vi "CAEN PSM SMART HV.vi"() -> ()   [LabVIEW 2017]
uses:
  <instrlib>/CAEN PSM/CAEN PSM.lvlib
panel:
  out "Output values":string[](array[string])
  in  "Value":string
  in  "mon button":bool
  in  "set button":bool
  out "Parameter descriptor":T1
  in  "info button":bool
  out "Connection status":bool
  in  "stop":bool
  in  "OK Button":bool
  out "error out":errorcluster
  in  "Tab Control":enum32{"Board", "Channel"}(tab)
  in  "Board Parameter":string(combo)
  in  "all_ch":bool
  in  "Channel number":u8
  in  "Channel Parameter":string(combo)
  out "Channel Parameters list":string[](array[string])
  out "Board Parameters list":string[](array[string])
  out "Module Info":T2
  in  "VISA resource name":refnum<visa-resource-name>
  # "CAEN PSM for the SMART HV devices\nVI example"
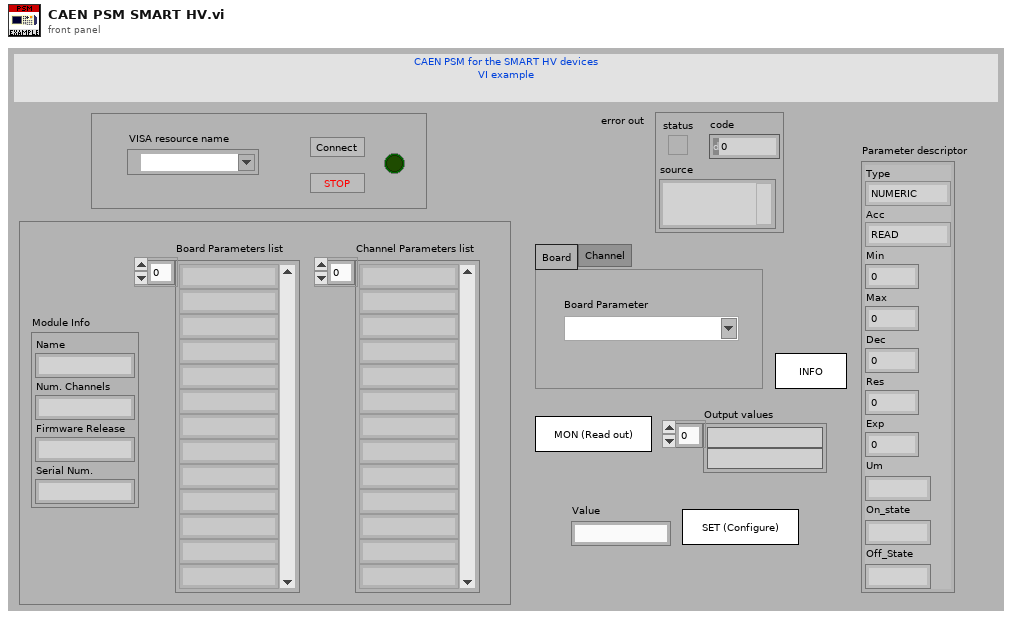
[diagram p1: front panel]
types:
  T1 = cluster{"Type":enum16{"NUMERIC", "ONOFF", "CHSTATUS", "BDSTATUS", "BINARY", "STRING", "ENUM"}, "Acc":enum16{"READ", "WRITE", "READ_WRITE"}, "Min":u32, "Max":u32, "Dec":u32, "Res":u32, "Exp":i32, "Um":string, "On_state":string, "Off_State":string}
  T2 = cluster{"Name":string, "Num. Channels":string, "Firmware Release":string, "Serial Num.":string}
  T3 = typedef "CAEN PSM.lvlib/BoardHandle.ctl" = cluster{"VISA resource name":refnum<visa-resource-name>, "Board address":i8, "NChannels":u8}
  T4 = enum8{"Enabled", "Disabled", "Disabled and Grayed Out"}
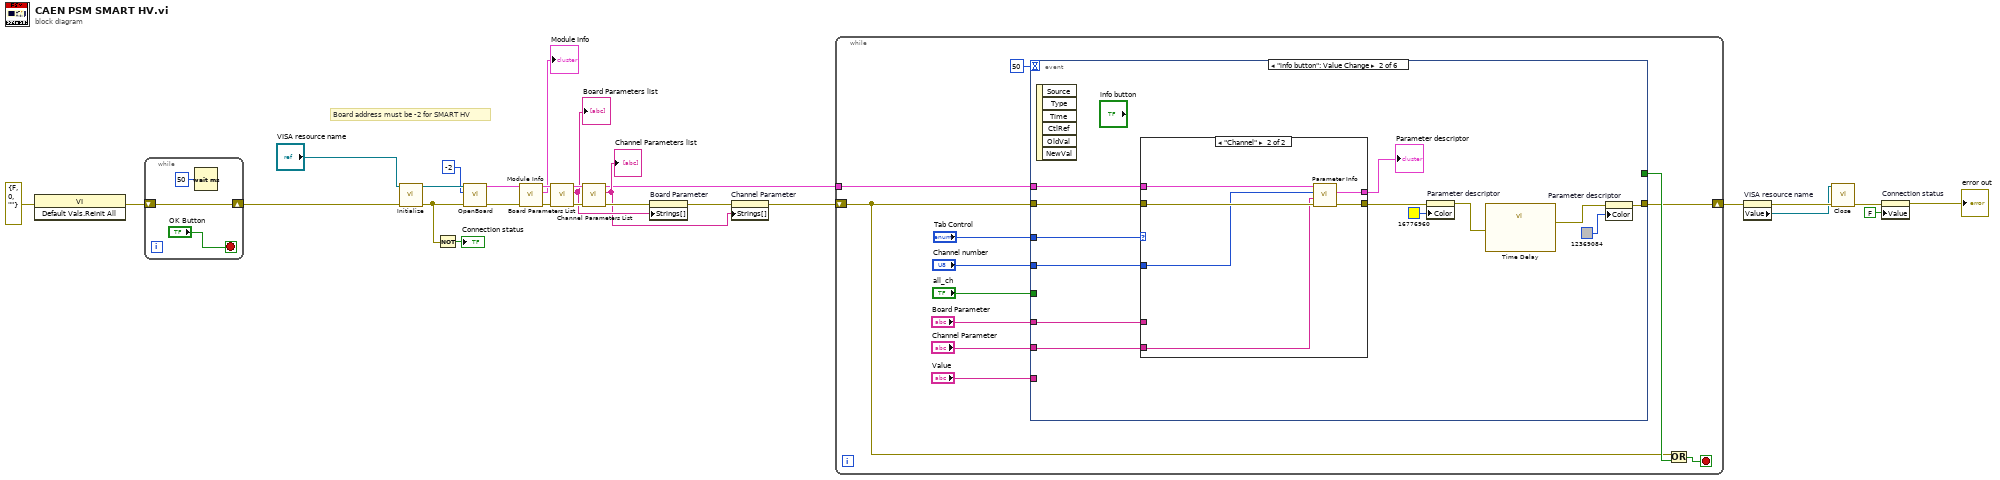
[diagram p0: block diagram]
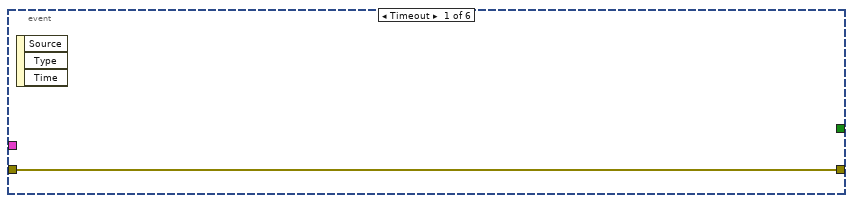
[diagram p2: hidden frame]
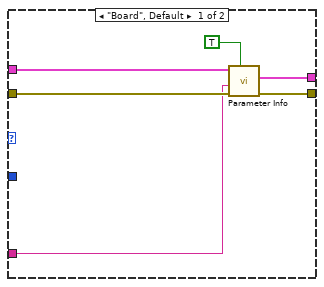
[diagram p3: hidden frame]
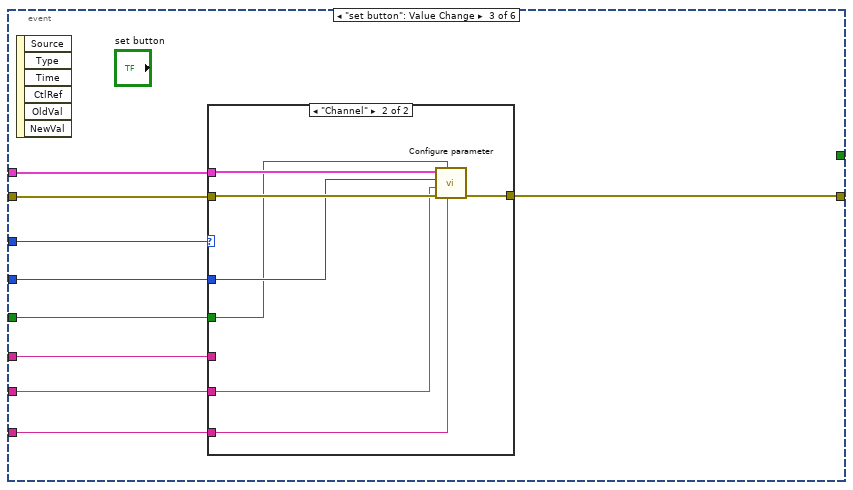
[diagram p4: hidden frame]
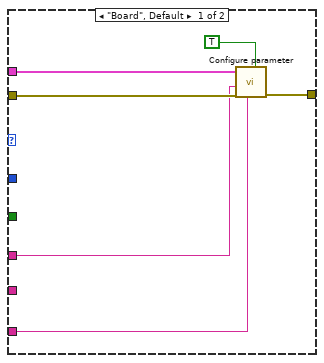
[diagram p5: hidden frame]
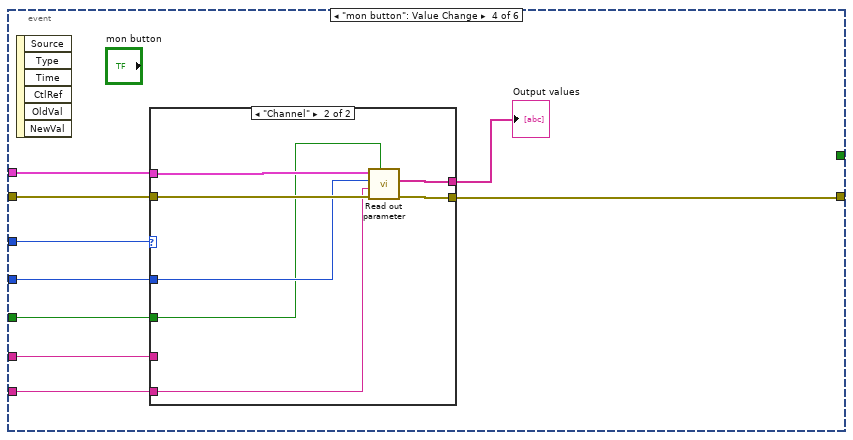
[diagram p6: hidden frame]
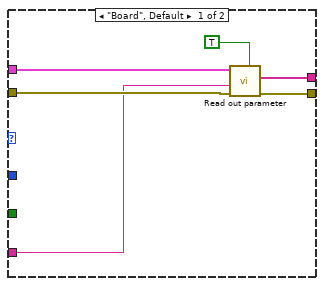
[diagram p7: hidden frame]
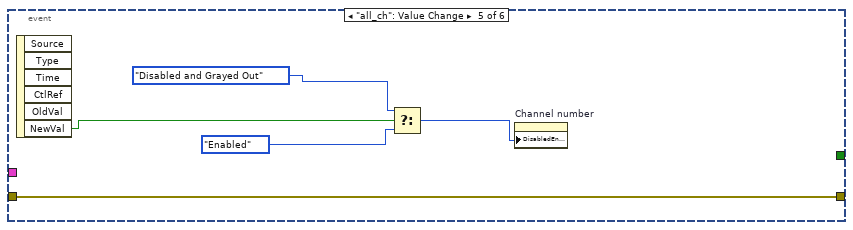
[diagram p8: hidden frame]
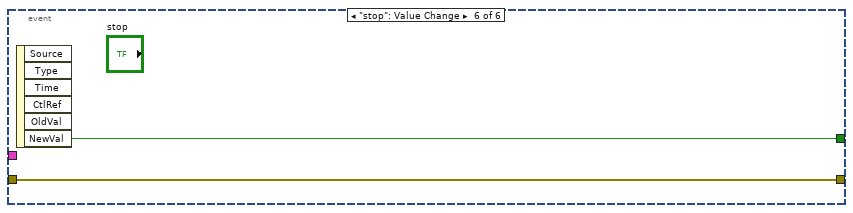
[diagram p9: hidden frame]
diagram:
  # "Board address must be -2 for SMART HV"
  n1 = invoke on="Invoke Node" class="VI" method="Default Vals.Reinit All"(error in=errorcluster {"status"=FALSE, "code"=0, "source"=""} ("error in (no error)")) -> (error out=w11:errorcluster)  [unwired: 2 in, 2 out]
  n2 = while {
    shift-right: [w30] -> w12
    shift-left: w11 -> [w30]
    stop <- "OK Button" stop-if-true
    n3 = Wait (ms)(milliseconds to wait=u32 50) -> ()  [unwired: 1 out]
  }
  n4 = call <instrlib>:"Initialize.vi"("error in (no error)"=w12, "VISA resource name"="VISA resource name") -> ("error out"=w8:errorcluster, "VISA resource name out"=w26:refnum<visa-resource-name>)  [unwired: 8 in]
  n5 = Not(x=w8) -> (.not. x?=→"Connection status":bool)
  n6 = call <instrlib>:"OpenBoard.vi"("error in (no error)"=w8, "Board Address"=i8 -2, "VISA resource name"=w26) -> ("error out"=w9:errorcluster, "BoardHandle"=w24:T3)  [unwired: 7 in]
  n7 = call <instrlib>:"Module Info.vi"("error in (no error)"=w9, "BoardHandle"=w24) -> ("error out"=w23:errorcluster, "Module Info"=→"Module Info":T2, "BoardHandle out"=w21:T3)  [unwired: 7 in]
  n8 = call <instrlib>:"Board Parameters List.vi"("error in (no error)"=w23, "BoardHandle"=w21) -> ("error out"=w22:errorcluster, "Parameters list"=w14:string[], "BoardHandle out"=w19:T3)  [unwired: 6 in, 1 out]
  "Board Parameters list" <- w14
  n9 = call <instrlib>:"Channel Parameters List.vi"("error in (no error)"=w22, "BoardHandle"=w19) -> ("error out"=w16:errorcluster, "Parameters list"=w13:string[], "BoardHandle out"=w1:T3)  [unwired: 6 in, 1 out]
  "Channel Parameters list" <- w13
  n10 = property on="Board Parameter" class="CmbBox"(error in=w16, "Strings[]"=w14) -> (error out=w15:errorcluster)  [unwired: 1 in, 1 out]
  n11 = property on="Channel Parameter" class="CmbBox"(error in=w15, "Strings[]"=w13) -> (error out=w6:errorcluster)  [unwired: 1 in, 1 out]
  n12 = while {
    shift-right: [w39] -> w5
    shift-left: w6 -> [w40]
    tunnel: w1 -> [w37]
    stop <- w42 stop-if-true
    n13 = event shown="[1] \"info button\": Value Change" {
      selector: _ -> [_ _ _ _ _ _]
      dyn-events: _ -> [_ _ _ _ _ _]
      timeout: 50 -> [_ _ _ _ _ _]
      tunnel: [_ _ _ _ _ w119] -> w41
      tunnel: w40 -> [w43 w56 w77 w98 w113 w118]
      tunnel: [w43 w47 w76 w97 w113 w118] -> w39
      tunnel: w37 -> [_ w55 w75 w99 _ _]
      tunnel: "Tab Control" -> [_ w53 w69 w94 _ _]
      tunnel: "Channel number" -> [_ w50 w71 w93 _ _]
      tunnel: "all_ch" -> [_ _ w70 w91 _ _]
      tunnel: "Board Parameter" -> [_ w52 w74 w95 _ _]
      tunnel: "Channel Parameter" -> [_ w51 w72 w92 _ _]
      tunnel: "Value" -> [_ _ w73 _ _ _]
      event Timeout {
        n14 = event-data() -> ()  [unwired: 1 in, 3 out]
      }
      event "info button": Value Change {
        n15 = event-data() -> ()  [unwired: 1 in, 6 out]
        n16 = case shown="\"Channel\"" w53 {
          tunnel: w56 -> [w62 w68]
          tunnel: w55 -> [w59 w67]
          tunnel: [w61 w66] -> w49
          tunnel: [w60 w65] -> w54
          tunnel: w52 -> [w57 _]
          tunnel: w51 -> [_ w64]
          tunnel: w50 -> [_ w63]
          frame "Board", Default {
            n17 = call <instrlib>:"Parameter Info.vi"("Board parameter? (F)"=TRUE, "error in (no error)"=w62, "Parameter name"=w57, "BoardHandle"=w59) -> ("error out"=w61:errorcluster, "Parameter descriptor"=w60:T1)  [unwired: 5 in, 1 out]
          }
          frame "Channel" {
            n18 = call <instrlib>:"Parameter Info.vi"("error in (no error)"=w68, "Parameter name"=w64, "Channel"=w63, "BoardHandle"=w67) -> ("error out"=w66:errorcluster, "Parameter descriptor"=w65:T1)  [unwired: 5 in, 1 out]
          }
        }
        "Parameter descriptor" <- w54
        n19 = property on="Parameter descriptor" class="Clust (strict)"(error in=w49, "Color"=u32 16776960) -> (error out=w48:errorcluster)  [unwired: 1 in, 1 out]
        n20 = call "Time Delay"("error in (no error)"=w48) -> ("error out"=w46:errorcluster)  [unwired: 10 in]
        n21 = property on="Parameter descriptor" class="Clust (strict)"(error in=w46, "Color"=u32 12369084) -> (error out=w47:errorcluster)  [unwired: 1 in, 1 out]
      }
      event "set button": Value Change {
        n22 = event-data() -> ()  [unwired: 1 in, 6 out]
        n23 = case shown="\"Channel\"" w69 {
          tunnel: w77 -> [w83 w89]
          tunnel: [w82 w90] -> w76
          tunnel: w75 -> [w81 w85]
          tunnel: w74 -> [w79 _]
          tunnel: w73 -> [w78 w87]
          tunnel: w72 -> [_ w88]
          tunnel: w71 -> [_ w86]
          tunnel: w70 -> [_ w84]
          frame "Board", Default {
            n24 = call <instrlib>:"Configure parameter.vi"("Board parameter? (F)"=TRUE, "String value"=w78, "error in (no error)"=w83, "Parameter name"=w79, "BoardHandle"=w81) -> ("error out"=w82:errorcluster)  [unwired: 5 in, 1 out]
          }
          frame "Channel" {
            n25 = call <instrlib>:"Configure parameter.vi"("String value"=w87, "All Channels (F)"=w84, "error in (no error)"=w89, "Parameter name"=w88, "Channel (0)"=w86, "BoardHandle"=w85) -> ("error out"=w90:errorcluster)  [unwired: 4 in, 1 out]
          }
        }
      }
      event "mon button": Value Change {
        n26 = event-data() -> ()  [unwired: 1 in, 6 out]
        n27 = case shown="\"Channel\"" w94 {
          tunnel: w99 -> [w105 w110]
          tunnel: w98 -> [w104 w109]
          tunnel: [w103 w112] -> w97
          tunnel: [w102 w111] -> w96
          tunnel: w95 -> [w100 _]
          tunnel: w93 -> [_ w108]
          tunnel: w92 -> [_ w107]
          tunnel: w91 -> [_ w106]
          frame "Board", Default {
            n28 = call <instrlib>:"Read out parameter.vi"("Board parameter? (F)"=TRUE, "error in (no error)"=w104, "Parameter name"=w100, "BoardHandle"=w105) -> ("error out"=w103:errorcluster, "Output values"=w102:string[])  [unwired: 5 in, 1 out]
          }
          frame "Channel" {
            n29 = call <instrlib>:"Read out parameter.vi"("All Channels (F)"=w106, "error in (no error)"=w109, "Parameter name"=w107, "Channel"=w108, "BoardHandle"=w110) -> ("error out"=w112:errorcluster, "Output values"=w111:string[])  [unwired: 4 in, 1 out]
          }
        }
        "Output values" <- w96
      }
      event "all_ch": Value Change {
        n30 = event-data() -> ("NewVal"=w115:bool)  [unwired: 1 in, 5 out]
        n31 = Select(t=T4."Disabled and Grayed Out" ("Disabled"), s=w115, f=T4."Enabled" ("Disabled")) -> (s? t:f=w114:T4)
        n32 = property on="Channel number" class="DigNum (strict)"("DisabledEnum"=w114) -> ()  [unwired: 2 in, 2 out]
      }
      event "stop": Value Change {
        n33 = event-data() -> ("NewVal"=w119:bool)  [unwired: 1 in, 5 out]
      }
    }
    n34 = Or(x=w40, y=w41) -> (x .or. y?=w42:bool)
  }
  n35 = property on="VISA resource name" class="VISAName"(error in=w5) -> (error out=w18:errorcluster, "Value"=w17:refnum<visa-resource-name>)  [unwired: 1 in, 1 out]
  n36 = call <instrlib>:"Close.vi"("error in (no error)"=w18, "VISA resource name"=w17) -> ("error out"=w4:errorcluster)  [unwired: 9 in]
  n37 = property on="Connection status" class="Bool (strict)"(error in=w4, "Value"=FALSE ("Connection status")) -> (error out=→"error out":errorcluster)  [unwired: 1 in, 1 out]
